vi "traj_coe_write_CPT.vi"() -> ()   [LabVIEW 2014]
uses:
  <vilib>/Utility/file.llb/Read From Spreadsheet File (DBL).vi
  <vilib>/FPGAPlugInAG/cRIO-9066/niLvFpga_Open_cRIO-9066.vi
  <vilib>/Utility/error.llb/Error Cluster From Error Code.vi
  <vilib>/rvi/errors/niLvFpgaAdjustHostInterfaceError.vi
  <vilib>/rvi/interface/nirviOpenFPGA/nirviOpenFPGA.xnode
  FPGA Bitfiles/forcecontroledu_FPGATarget_CPTread_lsxOFgf5HFo.lvbitx
  <vilib>/rvi/interface/nirviMethod/nirviMethod.xnode
  <vilib>/rvi/errors/niLvFpgaMergeErrorWithErrorCode.vi
  <vilib>/FPGAPlugInAG/cRIO-9066/niLvFpga_StartFifo_cRIO-9066.vi
  <vilib>/FPGAPlugInAG/cRIO-9066/niLvFpga_WriteFifo_cRIO-9066.vi
panel:
  out "A3":dbl[](array[numeric]) format="%.2f"
  out "writing_done":bool
  in  "stop":bool
  out "A1":dbl[](array[numeric]) format="%.2f"
  out "A2":dbl[](array[numeric]) format="%.2f"
  out "A0":dbl[](array[numeric]) format="%.2f"
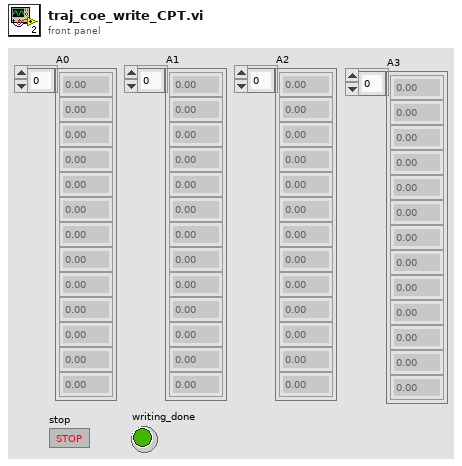
[diagram p1: front panel]
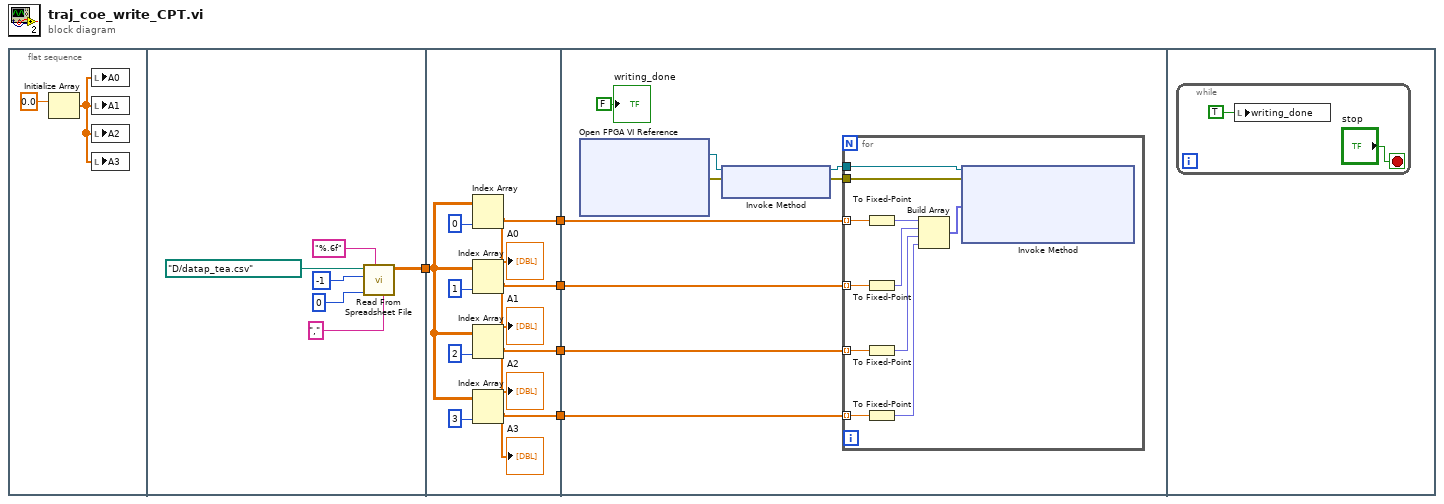
[diagram p0: block diagram]
diagram:
  n1 = flat-sequence {
    tunnel: [w8] -> w5
    tunnel: w5 -> [w15]
    tunnel: [w19] -> w4
    tunnel: [w18] -> w3
    tunnel: [w17] -> w2
    tunnel: [w14] -> w1
    tunnel: w4 -> [w27]
    tunnel: w3 -> [w26]
    tunnel: w2 -> [w25]
    tunnel: w1 -> [w23]
    frame #0 {
      n2 = Initialize Array(0.0 ("element")) -> (w6:dbl[])  [unwired: 1 in]
      n3 = local write "A0"(w6) -> ()
      n4 = local write "A1"(w6) -> ()
      n5 = local write "A2"(w6) -> ()
      n6 = local write "A3"(w6) -> ()
    }
    frame #1 {
      n7 = call-poly <vilib>:"Read From Spreadsheet File.vi"("delimiter (\\t)"="," ("delimiter (\\t)"), "format (%.3f)"="%.6f" ("format (%d)"), "max characters/row  (no limit:0)"=0, "number of rows (all:-1)"=-1, "file path (dialog if empty)"=path "D:/datap_tea.csv") -> ("all rows"=w8:dbl[][])  [unwired: 2 in, 4 out]
    }
    frame #2 {
      n8 = Index Array(array=w15, index (col)=0 ("disabled index (col)")) -> (element=w19:dbl[])  [unwired: 1 in]
      "A0" <- w19
      n9 = Index Array(array=w15, index (col)=1 ("disabled index (col)")) -> (element=w18:dbl[])  [unwired: 1 in]
      "A1" <- w18
      n10 = Index Array(array=w15, index (col)=2 ("disabled index (col)")) -> (element=w17:dbl[])  [unwired: 1 in]
      "A2" <- w17
      n11 = Index Array(array=w15, index (col)=3 ("disabled index (col)")) -> (element=w14:dbl[])  [unwired: 1 in]
      "A3" <- w14
    }
    frame #3 {
      n12 = xnode "Open FPGA VI Reference"() -> ("FPGA VI Reference Out"=w31:refnum<k20>, "error out"=w30:errorcluster)  [unwired: 2 in]
      n13 = xnode "Invoke Method"("FPGA VI Reference In"=w31, "error in"=w30) -> ("FPGA VI Reference Out"=w29:refnum<k20>, "error out"=w28:errorcluster)
      n14 = for {
        tunnel: w29 -> [w34]
        tunnel: w28 -> [w33]
        tunnel: w27 -> [w42] mode=indexing
        tunnel: w26 -> [w41] mode=indexing
        tunnel: w25 -> [w40] mode=indexing
        tunnel: w23 -> [w36] mode=indexing
        n15 = To Fixed-Point(number=w42) -> (fixed-point=w39:fxp<+/-,55,35>)  [unwired: 1 in]
        n16 = To Fixed-Point(number=w41) -> (fixed-point=w38:fxp<+/-,55,35>)  [unwired: 1 in]
        n17 = To Fixed-Point(number=w40) -> (fixed-point=w37:fxp<+/-,55,35>)  [unwired: 1 in]
        n18 = To Fixed-Point(number=w36) -> (fixed-point=w35:fxp<+/-,55,35>)  [unwired: 1 in]
        n19 = Build Array(w39, w38, w37, w35) -> (w32:fxp<+/-,55,35>[])
        n20 = xnode "Invoke Method"("FPGA VI Reference In"=w34, "error in"=w33, "Data"=w32) -> ()  [unwired: 1 in, 3 out]
      }
      "writing_done" <- FALSE ("writing_done")
    }
    frame #4 {
      n21 = while {
        stop <- "stop" stop-if-true
        n22 = local write "writing_done"(TRUE ("writing_done")) -> ()
      }
    }
  }
